vi "Initialize.vi"(8 "error in (no error)":errorcluster, 9 "Send \"Connect client\"":bool=TRUE, 10 "Reset":bool=TRUE, 11 "RP Instrument in":refnum<class "RP Instrument.lvclass">) -> (0 "error out":errorcluster, 3 "RP Instrument out":refnum<class "RP Instrument.lvclass">)   [LabVIEW 2016, in "RP Instrument.lvclass"]
uses:
  RP Instrument.lvclass
  RP Command.ctl
  RP Config Offsets.ctl
  RP Instrument.lvclass/RP Instrument.ctl
  RP Communicator/RP Communicator.lvclass
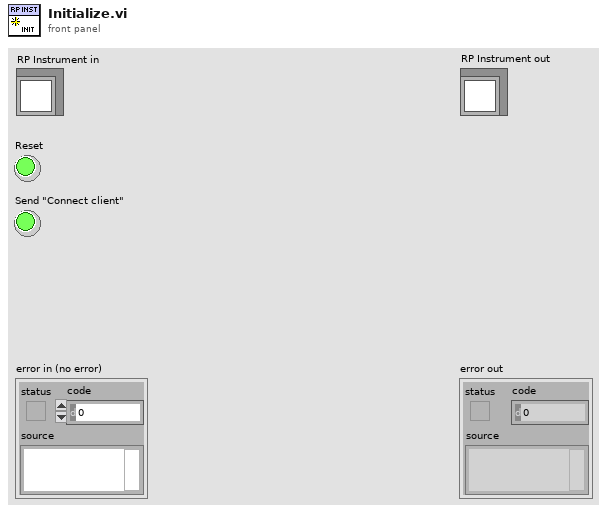
[diagram p1: front panel]
types:
  T1 = typedef "RP Command.ctl" = enum16{"Reset", "Read IDN", "Stop server", "Get status", "Get temperature", "Connect client", "Arm", "Software trigger", "Get whole buffer", "Get chunk", "System call", "Get config", "Set config", "Recieve data", "Play pattern", "Transmit data"}
  T2 = typedef "RP Config Offsets.ctl" = u16
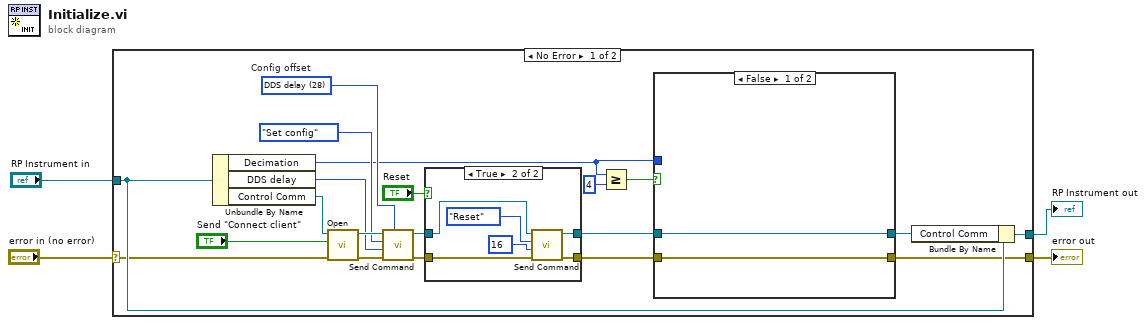
[diagram p0: block diagram]
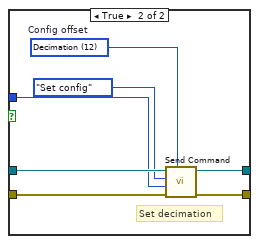
[diagram p2: hidden frame]
diagram:
  n1 = case shown="No Error" "error in (no error)" {
    selector: "error in (no error)" -> [w22 w43]
    tunnel: [w18 w43] -> w3
    tunnel: [w21 w42] -> w1
    tunnel: "RP Instrument in" -> [w24 w42]
    frame No Error {
      w9 = T2 28 items=["Config flags"=0, "Record length"=4, "Frequency"=8, "Decimation"=12, "LED"=16, "DDS delay"=28]  # Config offset
      n2 = Unbundle By Name(w24) -> ("Decimation"=w7:u32, "DDS delay"=w10:u32, "Control Comm"=w23:refnum<class "RP Communicator.lvclass">)
      n3 = call-dynamic "Open.vi"("error in (no error)"=w22, "Send \"Connect client\""="Send \"Connect client\"", "RP Communicator in"=w23) -> ("error out"=w12:errorcluster, "RP Communicator out"=w13:refnum<class "RP Communicator.lvclass">)  [unwired: 7 in]
      n4 = call-dynamic "Send Command.vi"("Config offset"=w9, "error in (no error)"=w12, "Command payload"=w10, "Command number"=RP_Command."Set config", "RP Communicator in"=w13) -> ("error out"=w15:errorcluster, "RP Communicator out"=w14:refnum<class "RP Communicator.lvclass">)  [unwired: 5 in]
      n5 = case shown="True" "Reset" {
        tunnel: [w34 w39] -> w20
        tunnel: w15 -> [w34 w38]
        tunnel: w14 -> [w35 w37]
        tunnel: [w35 w36] -> w19
        frame False {
        }
        frame True {
          n6 = call-dynamic "Send Command.vi"("error in (no error)"=w38, "Command payload"=u64 16, "Command number"=RP_Command."Reset", "RP Communicator in"=w37) -> ("error out"=w39:errorcluster, "RP Communicator out"=w36:refnum<class "RP Communicator.lvclass">)  [unwired: 6 in]
        }
      }
      n7 = Greater Or Equal?(x=w7, y=u32 4) -> (x >= y?=w5:bool)
      n8 = case shown="False" w5 {
        tunnel: w20 -> [w25 w33]
        tunnel: w19 -> [w26 w32]
        tunnel: [w25 w31] -> w18
        tunnel: [w26 w30] -> w17
        tunnel: w7 -> [_ w29]
        frame False {
        }
        frame True {
          w28 = T2 12 items=["Config flags"=0, "Record length"=4, "Frequency"=8, "Decimation"=12, "LED"=16]  # Config offset
          # "Set decimation"
          n9 = call-dynamic "Send Command.vi"("Config offset"=w28, "error in (no error)"=w33, "Command payload"=w29, "Command number"=RP_Command."Set config", "RP Communicator in"=w32) -> ("error out"=w31:errorcluster, "RP Communicator out"=w30:refnum<class "RP Communicator.lvclass">)  [unwired: 5 in]
        }
      }
      n10 = Bundle By Name(cluster=w24, "Control Comm"=w17) -> (w21:refnum<class "RP Instrument.lvclass">)
    }
    frame Error {
    }
  }
  "error out" <- w3
  "RP Instrument out" <- w1
